vi "Test11.vi"() -> ()   [LabVIEW 2010]
uses:
  <vilib>/MDSplus/Library/MDSplus.lvlib
panel:
  in  "Path":string=":NUMX"
  in  "Mode":string="EDIT"
  in  "Shot":i32=-1
  in  "Name":string="my_tree"
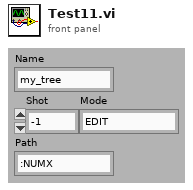
[diagram p1: front panel]
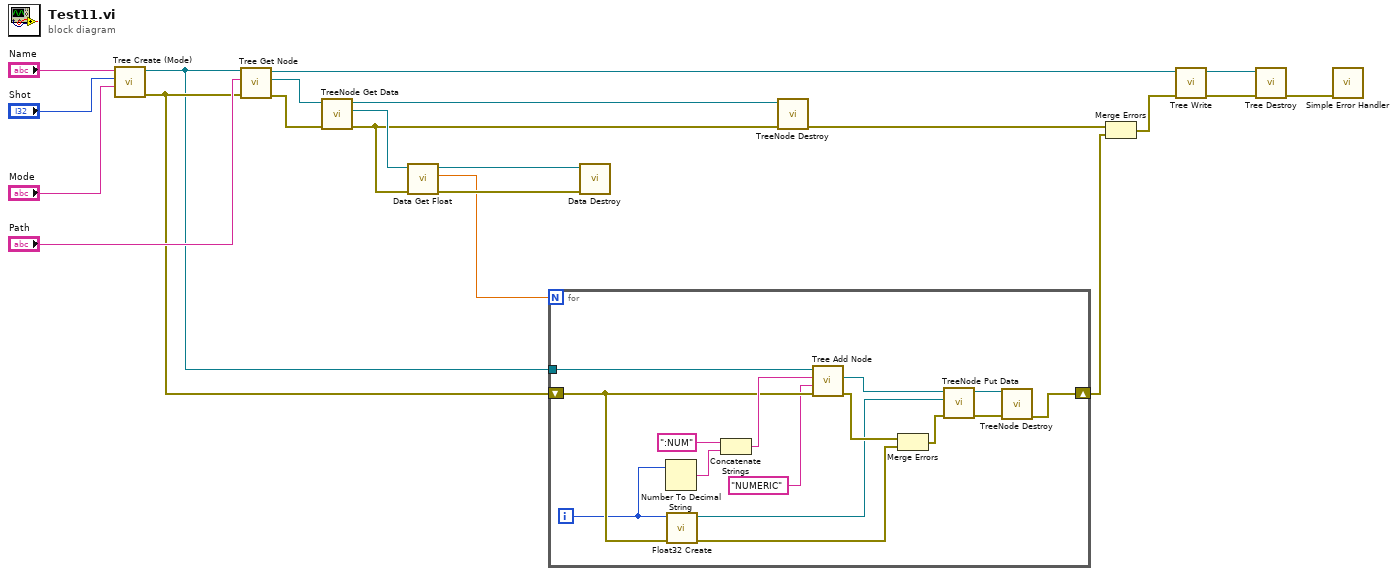
[diagram p0: block diagram]
diagram:
  n1 = call <vilib>:"Tree Create (Mode).vi"("Mode"="Mode", "Shot"="Shot", "Name"="Name") -> ("error out"=w13:errorcluster, "Tree DVR out"=w12:refnum<data-value>)  [unwired: 7 in]
  n2 = call <vilib>:"Tree Get Node.vi"("error in (no error)"=w13, "Path"="Path", "Tree DVR in"=w12) -> ("error out"=w15:errorcluster, "Node out"=w17:refnum<data-value>, "Tree DVR out"=w5:refnum<data-value>)  [unwired: 6 in]
  n3 = call <vilib>:"TreeNode Get Data.vi"("error in (no error)"=w15, "TreeNode DVR in"=w17) -> ("error out"=w6:errorcluster, "Data out"=w16:refnum<data-value>, "TreeNode DVR out"=w7:refnum<data-value>)  [unwired: 7 in]
  n4 = call <vilib>:"Data Get Float.vi"("error in (no error)"=w6, "Data DVR in"=w16) -> ("error out"=w14:errorcluster, "SGL out"=w8:sgl, "Data DVR out"=w1:refnum<data-value>)  [unwired: 7 in]
  n5 = for {
    N: w8 -> [_]
    tunnel: w12 -> [w34]
    shift-right: [w27] -> w11
    shift-left: w13 -> [w26]
    i -> [w25]
    n6 = Number To Decimal String(number=w25) -> (decimal integer string=w35:string)  [unwired: 1 in]
    n7 = call <vilib>:"Float32 Create.vi"("error in (no error)"=w26, "SGL in"=w25) -> ("error out"=w31:errorcluster, "Float32 DVR out"=w22:refnum<data-value>)  [unwired: 8 in]
    n8 = Concatenate Strings(":NUM", w35) -> (w33:string)
    n9 = call <vilib>:"Tree Add Node.vi"("error in (no error)"=w26, "Usage"="NUMERIC", "Name"=w33, "Tree DVR in"=w34) -> ("error out"=w30:errorcluster, "Node out"=w23:refnum<data-value>)  [unwired: 5 in, 1 out]
    n10 = Merge Errors(w30, w31) -> (w32:errorcluster)
    n11 = call <vilib>:"TreeNode Put Data.vi"("error in (no error)"=w32, "Data"=w22, "TreeNode DVR in"=w23) -> ("error out"=w28:errorcluster, "TreeNode DVR out"=w29:refnum<data-value>)  [unwired: 7 in]
    n12 = call <vilib>:"TreeNode Destroy.vi"("error in (no error)"=w28, "TreeNode DVR in"=w29) -> ("error out"=w27:errorcluster)  [unwired: 9 in]
  }
  n13 = call <vilib>:"Data Destroy.vi"("error in (no error)"=w14, "Data DVR in"=w1) -> ()  [unwired: 9 in, 1 out]
  n14 = call <vilib>:"TreeNode Destroy.vi"("error in (no error)"=w6, "TreeNode DVR in"=w7) -> ("error out"=w10:errorcluster)  [unwired: 9 in]
  n15 = Merge Errors(w10, w11) -> (w3:errorcluster)
  n16 = call <vilib>:"Tree Write.vi"("error in (no error)"=w3, "Tree DVR in"=w5) -> ("error out"=w2:errorcluster, "Tree DVR out"=w4:refnum<data-value>)  [unwired: 8 in]
  n17 = call <vilib>:"Tree Destroy.vi"("error in (no error)"=w2, "Tree DVR in"=w4) -> ("error out"=w9:errorcluster)  [unwired: 9 in]
  n18 = call <vilib>:"Simple Error Handler.vi"("error in (no error)"=w9) -> ()  [unwired: 4 in, 5 out]
